vi "CC Convert RA to String.vi"(8 "error in (no error)":errorcluster, 11 "RA":dbl) -> (0 "error out":errorcluster, 2 "Right Ascension":T1, 3 "RA String":string)   [LabVIEW 2021]
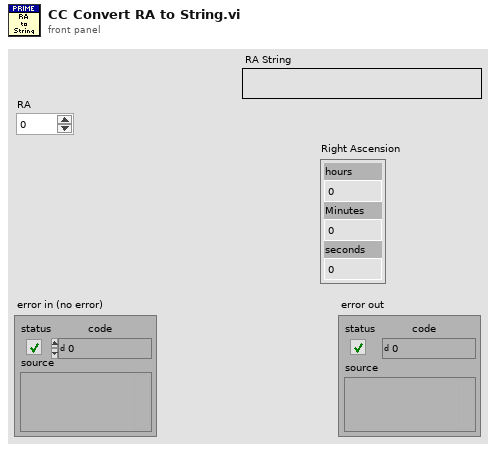
[diagram p1: front panel]
types:
  T1 = cluster{"hours":dbl, "Minutes":dbl, "seconds":dbl}
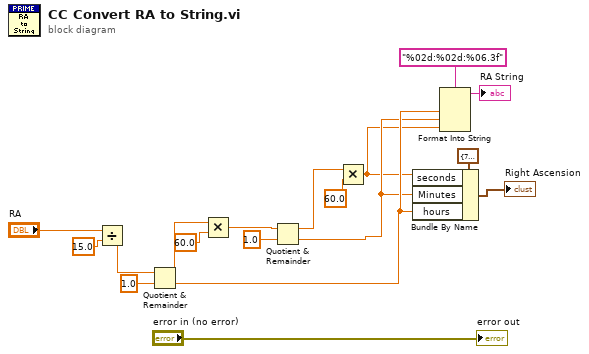
[diagram p0: block diagram]
diagram:
  n1 = Divide(x="RA", y=15.0) -> (x/y=w14:dbl)
  n2 = Quotient & Remainder(x=w14, y=1.0) -> (x-y*floor(x/y)=w12:dbl, floor(x/y)=w5:dbl)
  n3 = Multiply(x=w12, y=60.0) -> (x*y=w11:dbl)
  n4 = Quotient & Remainder(x=w11, y=1.0) -> (x-y*floor(x/y)=w10:dbl, floor(x/y)=w4:dbl)
  n5 = Multiply(x=w10, y=60.0) -> (x*y=w3:dbl)
  n6 = Bundle By Name(cluster=T1 {"hours"=7.0, "Minutes"=57.0, "seconds"=16.79999999999879} ("Degrees"), "seconds"=w3, "Minutes"=w4, "hours"=w5) -> (→"Right Ascension":T1)
  n7 = Format Into String(format string="%02d:%02d:%06.3f", w5, w4, w3) -> (resulting string=→"RA String":string)  [unwired: 2 in, 1 out]
  "error out" <- "error in (no error)"
